vi "Select File.vi"(8 "error in (no error)":errorcluster, 10 "Mode":T1(ring), 11 "TIFF in":refnum<class "TIFF.lvclass">) -> (0 "error out":errorcluster, 3 "TIFF out":refnum<class "TIFF.lvclass">)   [LabVIEW 2018, in "BinaryTIFF.lvlib" / "TIFF.lvclass"]
uses:
  TIFF.lvclass
  TIFF.lvclass/TIFF.ctl
  <vilib>/Utility/error.llb/Error Cluster From Error Code.vi
  <vilib>/ErrorRing/Error Ring.xnode
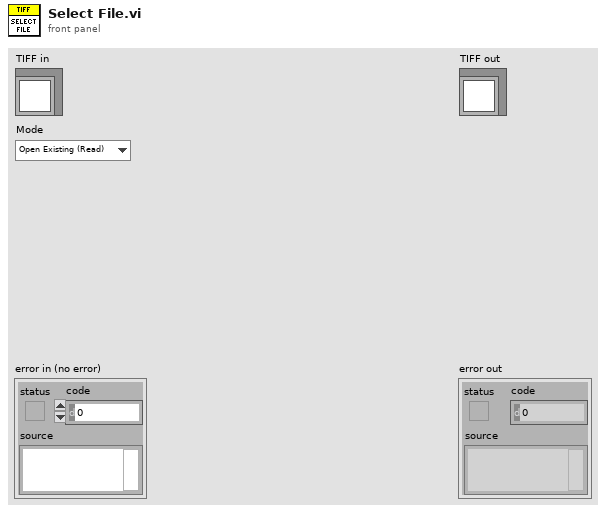
[diagram p1: front panel]
types:
  T1 = enum16{"Open Existing (Read)", "Create or Replace (Write)"}
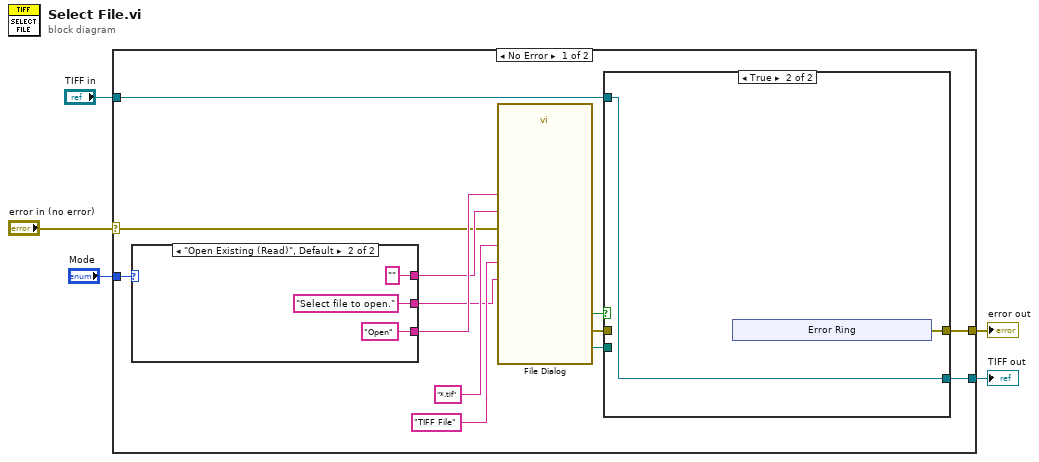
[diagram p0: block diagram]
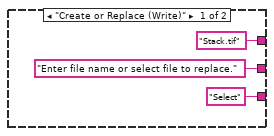
[diagram p2: hidden frame]
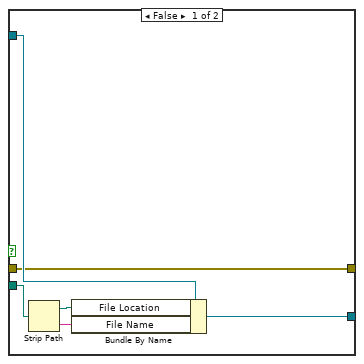
[diagram p3: hidden frame]
diagram:
  n1 = case shown="No Error" "error in (no error)" {
    selector: "error in (no error)" -> [w6 w38]
    tunnel: [w15 w38] -> w4
    tunnel: [w13 w37] -> w2
    tunnel: "TIFF in" -> [w14 w37]
    tunnel: "Mode" -> [w10 _]
    frame No Error {
      n2 = case shown="\"Open Existing (Read)\", Default" w10 {
        tunnel: ["Select" ("button label") "Open" ("button label")] -> w9
        tunnel: ["Stack.tif" ("button label") "" ("button label")] -> w8
        tunnel: ["Enter file name or select file to replace." ("button label") "Select file to open." ("button label")] -> w7
        frame "Create or Replace (Write)" {
        }
        frame "Open Existing (Read)", Default {
        }
      }
      n3 = call "File Dialog"("prompt"=w7, "button label"=w9, "default name"=w8, "error in"=w6, "pattern (all files)"="*.tif", "pattern label"="TIFF File") -> ("selected path"=w12:path, "cancelled"=w16:bool, "error out"=w11:errorcluster)  [unwired: 6 in, 1 out]
      n4 = case shown="True" w16 {
        tunnel: [w25 w31] -> w15
        tunnel: w14 -> [w30 w32]
        tunnel: [w29 w32] -> w13
        tunnel: w12 -> [w28 _]
        tunnel: w11 -> [w25 _]
        frame False {
          n5 = Strip Path(path=w28) -> (stripped path=w26:path, name=w27:string)
          n6 = Bundle By Name(cluster=w30, "File Location"=w26, "File Name"=w27) -> (w29:refnum<class "TIFF.lvclass">)
        }
        frame True {
          n7 = xnode "Error Ring"() -> ("error out"=w31:errorcluster)
        }
      }
    }
    frame Error {
    }
  }
  "error out" <- w4
  "TIFF out" <- w2
